vi "ANC300_trigger_setget.vi"(0 "ANC300 Communication Port In":refnum<visa-resource-name>, 1 "Axis":u8=1 min=1 max=7, 2 "Output - Up - Down":enum16{"Output", "Up", "Down"}(ring), 3 "Trigger Number - OFF":T3(ring), 4 "1 | 0 [only output trigger]":bool=TRUE, 5 "error in":T1, 6 "set | get":bool=TRUE, 7 "Time to wait [ms]":u32=200) -> (13 "command string":string, 14 "ANC300 Communication Port Out":refnum<visa-resource-name>, 15 "connection ID out":refnum<k5>, 16 "trigger status":string, 17 "Trigger Number - OFF":T2(ring), 18 "communication successful":cluster{bool, "read data":string}, 19 "error out":T1)   [LabVIEW 2012]
panel:
  out "transfer ok":bool
  out "data out":string
  in  "connection ID in":refnum<k5>
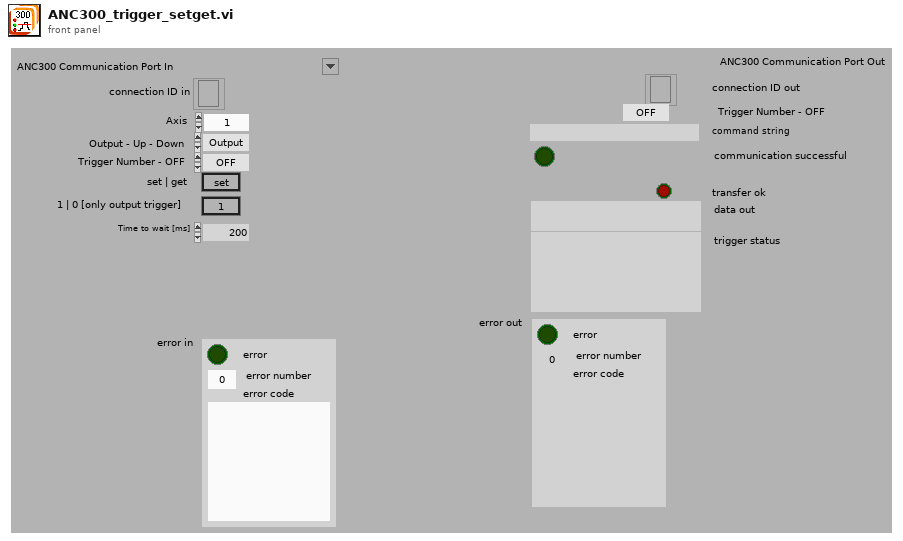
[diagram p1: front panel]
types:
  T1 = cluster{"error ":bool, "error number":i32, "error code":string}
  T2 = enum16{"OFF", "1", "2", "3", "4", "5", "6", "7", "8", "9", "10", "11", "12", "13", "14", "15", "16", "ERROR"}
  T3 = enum16{"OFF", "1", "2", "3", "4", "5", "6", "7", "8", "9", "10", "11", "12", "13", "14", "15", "16"}
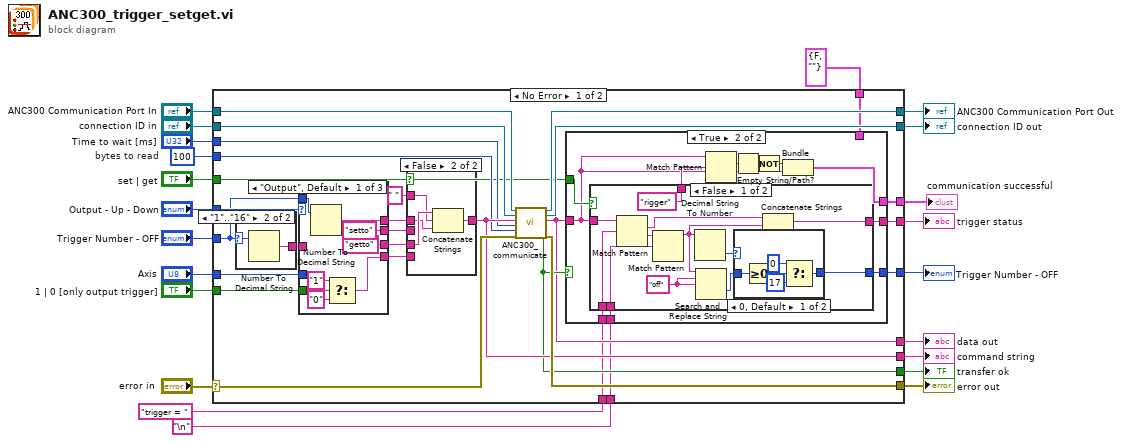
[diagram p0: block diagram]
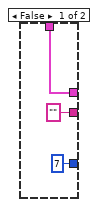
[diagram p2: hidden frame]
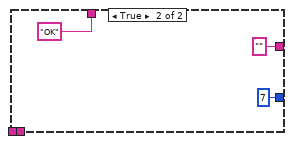
[diagram p4: hidden frame]
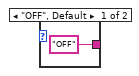
[diagram p5: hidden frame]
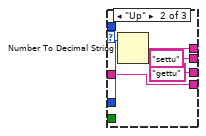
[diagram p6: hidden frame]
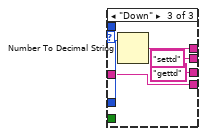
[diagram p7: hidden frame]
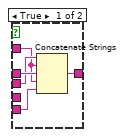
[diagram p8: hidden frame]
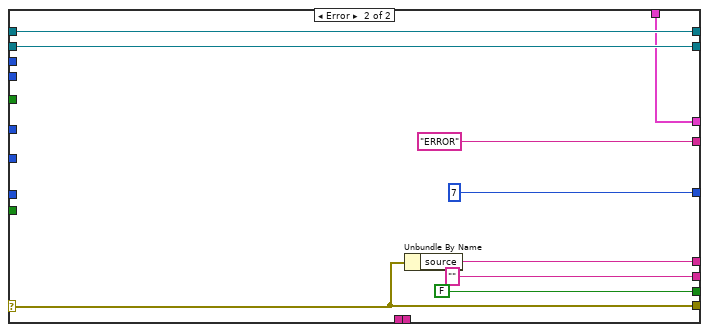
[diagram p9: hidden frame]
diagram:
  w13 = 100  # bytes to read
  n1 = case shown="No Error" "error in" {
    selector: "error in" -> [w40 w122]
    tunnel: "set | get" -> [w30 _]
    tunnel: "Output - Up - Down" -> [w50 _]
    tunnel: "Axis" -> [w48 _]
    tunnel: "Trigger Number - OFF" -> [w45 _]
    tunnel: "1 | 0 [only output trigger]" -> [w43 _]
    tunnel: "ANC300 Communication Port In" -> [w35 w124]
    tunnel: "connection ID in" -> [w36 w123]
    tunnel: "Time to wait [ms]" -> [w33 _]
    tunnel: w13 -> [w32 _]
    tunnel: [w38 w124] -> w12
    tunnel: [w37 w123] -> w11
    tunnel: [w39 w122] -> w3
    tunnel: [w31 FALSE ("transfer ok")] -> w10
    tunnel: [w34 ""] -> w9
    tunnel: [w29 w121] -> w8
    tunnel: "trigger = " -> [w28 _]
    tunnel: "\n" -> [w27 _]
    tunnel: [w26 "ERROR"] -> w5
    tunnel: [w25 7] -> w4
    tunnel: [w24 w116] -> w2
    tunnel: cluster{bool, "read data":string} {FALSE, "read data"=""} ("communication successful 2") -> [w23 w116]
    frame No Error {
      n2 = case shown="\"1\"..\"16\"" w45 {
        selector: w45 -> [_ w88]
        tunnel: ["OFF" w87] -> w49
        frame "OFF", Default {
        }
        frame "1".."16" {
          n3 = Number To Decimal String(number=w88) -> (decimal integer string=w87:string)  [unwired: 1 in]
        }
      }
      n4 = case shown="\"Output\", Default" w50 {
        tunnel: w49 -> [_ w97 w102]
        tunnel: w48 -> [_ w99 w103]
        tunnel: ["setto" "settu" "settd"] -> w47
        tunnel: ["getto" "gettu" "gettd"] -> w46
        tunnel: [w94 w98 w104] -> w44
        tunnel: w45 -> [w93 _ _]
        tunnel: w43 -> [w92 _ _]
        tunnel: [w89 w97 w102] -> w42
        frame "Output", Default {
          n5 = Number To Decimal String(number=w93) -> (decimal integer string=w94:string)  [unwired: 1 in]
          n6 = Select(t="1", s=w92, f="0") -> (s? t:f=w89:string)
        }
        frame "Up" {
          n7 = Number To Decimal String(number=w99) -> (decimal integer string=w98:string)  [unwired: 1 in]
        }
        frame "Down" {
          n8 = Number To Decimal String(number=w103) -> (decimal integer string=w104:string)  [unwired: 1 in]
        }
      }
      n9 = case shown="False" w30 {
        tunnel: w47 -> [w110 _]
        tunnel: w46 -> [_ w115]
        tunnel: w44 -> [w111 w114]
        tunnel: w42 -> [w109 _]
        tunnel: " " -> [w108 w113]
        tunnel: [w107 w112] -> w34
        frame True {
          n10 = Concatenate Strings(w110, w108, w111, w108, w109) -> (w107:string)
        }
        frame False {
          n11 = Concatenate Strings(w115, w113, w114) -> (w112:string)
        }
      }
      n12 = call "ANC300_communicate.vi"("ANC300 Communication Port In"=w35, "connection ID in"=w36, "commando string"=w34, "Time to wait [ms]"=w33, "bytes to read"=w32, "error in"=w40) -> ("ANC300 Communication Port Out"=w38:refnum<visa-resource-name>, "connection ID out"=w37:refnum<k5>, "read data"=w29:string, "transfer ok"=w31:bool, "error out"=w39:T1)  [unwired: 9 in]
      n13 = case shown="True" w31 {
        tunnel: w30 -> [_ w64]
        tunnel: w29 -> [_ w54]
        tunnel: w28 -> [_ w63]
        tunnel: w27 -> [_ w62]
        tunnel: ["" w61] -> w26
        tunnel: [7 w60] -> w25
        tunnel: [w51 w56] -> w24
        tunnel: w23 -> [w51 _]
        frame False {
        }
        frame True {
          n14 = case shown="False" w64 {
            tunnel: w54 -> [w69 _]
            tunnel: w63 -> [w76 _]
            tunnel: w62 -> [w74 _]
            tunnel: [w71 ""] -> w61
            tunnel: [w70 7] -> w60
            tunnel: ["rigger" "OK"] -> w55
            frame False {
              w65 = "off"
              n15 = Match Pattern(string=w69, regular expression=w76) -> (match substring=w72:string, after substring=w75:string)  [unwired: 1 in, 2 out]
              n16 = Match Pattern(string=w75, regular expression=w74) -> (before substring=w67:string)  [unwired: 1 in, 3 out]
              n17 = Decimal String To Number(string=w67) -> (number=w73:i32)  [unwired: 2 in, 1 out]
              n18 = Search and Replace String(input string=w67, search string=w65, replace string=w65) -> (offset past replacement=w66:i32)  [unwired: 5 in, 3 out]
              n19 = case shown="0, Default" w73 {
                selector: w73 -> [_ w82]
                tunnel: [w79 w82] -> w70
                tunnel: w66 -> [w77 _]
                frame 0, Default {
                  n20 = Greater Or Equal To 0?(x=w77) -> (x >= 0?=w78:bool)
                  n21 = Select(t=0, s=w78, f=17) -> (s? t:f=w79:i32)
                }
                frame 1..16 {
                }
              }
              n22 = Concatenate Strings(w72, w67) -> (w71:string)
            }
            frame True {
            }
          }
          n23 = Match Pattern(string=w54, regular expression=w55) -> (match substring=w57:string)  [unwired: 1 in, 3 out]
          n24 = Empty String/Path?(string/path=w57) -> (empty?=w58:bool)
          n25 = Not(x=w58) -> (.not. x?=w59:bool)
          n26 = Bundle(w59, "read data"=w54) -> (w56:cluster{bool, "read data":string})  [unwired: 1 in]
        }
      }
    }
    frame Error {
      n27 = Unbundle By Name(w122) -> ("source"=w121:string)
    }
  }
  "data out" <- w8
  "connection ID out" <- w11
  "command string" <- w9
  "transfer ok" <- w10
  "ANC300 Communication Port Out" <- w12
  "trigger status" <- w5
  "Trigger Number - OFF" <- w4
  "error out" <- w3
  "communication successful" <- w2
